vi "Turret_Control_Manual.vi"(1 "Rotate_Command":dbl) -> (0 "TurretMotorCommand":dbl)   [LabVIEW 2019]
uses:
  ArgosLib/ArgosLib.lvlib
panel:
  in  "Y_Array":dbl[](array[numeric])=[-1.0, 0.0, 0.0, 1.0] format="%.2f"
  in  "X_Array":dbl[](array[numeric])=[-1.0, -0.25, 0.25, 1.0] format="%.2f"
  in  "Max_Shooter_Rotate":dbl=0.5
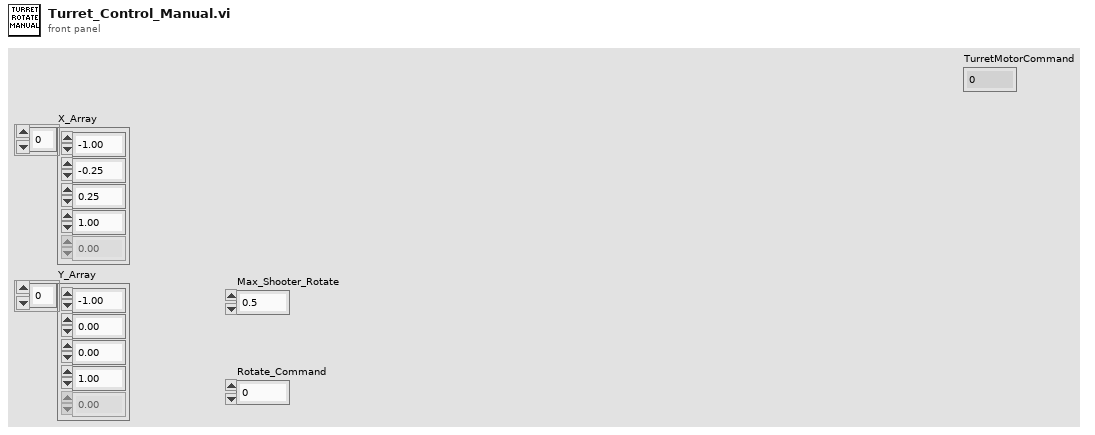
[diagram p1: front panel]
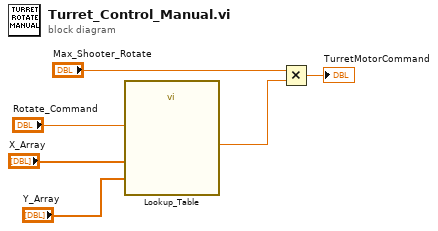
[diagram p0: block diagram]
diagram:
  n1 = call "Lookup_Table.vi"("Y_Array"="Y_Array", "x_in"="Rotate_Command", "X_Array"="X_Array") -> ("y_out"=w4:dbl)  [unwired: 6 in]
  n2 = Multiply(x="Max_Shooter_Rotate", y=w4) -> (x*y=→"TurretMotorCommand":dbl)
